vi "FourCornerAntennaComputePositionN.vi"(4 "y patch 1 position, mm":dbl=144.21 format="%.4f", 6 "x patch 1 position, mm":dbl=204.42 format="%.4f", 9 "y distance, mm":dbl format="%.4f", 10 "x distance, mm":dbl=83.143 format="%.4f", 11 "x direction angle, deg":dbl=0.295 format="%.4f") -> (2 "y":dbl, 3 "x":dbl)   [LabVIEW 2017]
doc: "Offsets x and y by the antenna #1 position to motion Home offset.\nCorrects x and y for rotation of the antenna wrt the motion frame of ref."
panel:
  # "corrected for antenna\nto motion frame \nangle offset"
  # "origin, offset from Home"
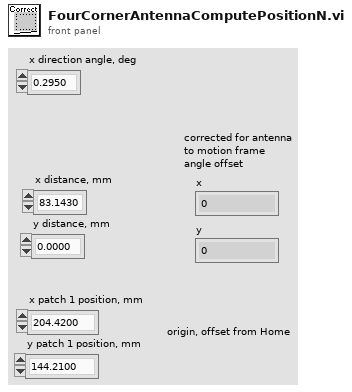
[diagram p1: front panel]
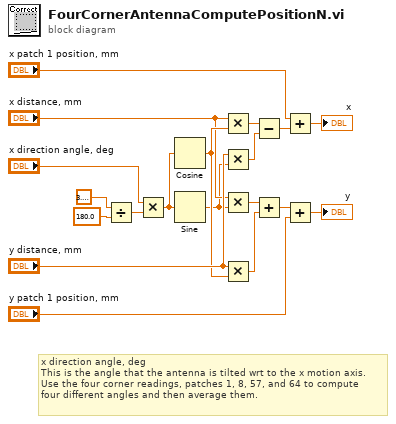
[diagram p0: block diagram]
diagram:
  # "x direction angle, deg\nThis is the angle that the antenna is tilted wrt to the x motion axis.\nUse the four corner readings, patches 1, 8, 57, and 64 to compute\nfour different angles and then average them."
  n1 = Divide(x=3.141592653589793, y=180.0) -> (x/y=w17:dbl)
  n2 = Multiply(x="x direction angle, deg", y=w17) -> (x*y=w14:dbl)
  n3 = Cosine(x=w14) -> (cos(x)=w10:dbl)
  n4 = Sine(x=w14) -> (sin(x)=w8:dbl)
  n5 = Multiply(x="x distance, mm", y=w10) -> (x*y=w15:dbl)
  n6 = Multiply(x="y distance, mm", y=w8) -> (x*y=w11:dbl)
  n7 = Multiply(x="x distance, mm", y=w8) -> (x*y=w7:dbl)
  n8 = Multiply(x="y distance, mm", y=w10) -> (x*y=w12:dbl)
  n9 = Subtract(x=w15, y=w11) -> (x-y=w6:dbl)
  n10 = Add(x=w7, y=w12) -> (x+y=w3:dbl)
  n11 = Add(x="x patch 1 position, mm", y=w6) -> (x+y=→"x":dbl)
  n12 = Add(x=w3, y="y patch 1 position, mm") -> (x+y=→"y":dbl)
